vi "Configure Trigger Layer.vi"(0 "VISA resource name":refnum<visa-resource-name>, 1 "Trigger Count (1)":i32=1, 2 "Trigger Source (0: Auto-Internal)":i32(ring) items=["Auto-Internal", "EXT1", "EXT2", "EXT3", "EXT4", "EXT5", "EXT6", "EXT7", "LAN", "Internal Bus 1", "Internal Bus 2", "Bus", "Timer"], 3 "Timer Trigger Interval (1E-4 s)":dbl=0.0001, 5 "Channel (1: Channel 1)":i32(ring)=1 items=["Channel 1"=1, "Channel 2"=2], 7 "Device Action (2: Both)":i32(ring)=2 items=["Acquire", "Transient", "Both"], 9 "Bypass Setting (0: Off)":i32(ring) items=["Off", "Once"], 11 "error in (no error)":errorcluster, 12 "Trigger Delay (0 s)":dbl, 13 "LXI Triggers For Normal Trigger":bool[](array[boolean])=[TRUE, TRUE, TRUE, TRUE, TRUE, TRUE, TRUE, TRUE]) -> (4 "VISA resource name out":refnum<visa-resource-name>, 15 "error out":errorcluster)   [LabVIEW 2012, in "Keysight B2980 Series.lvlib"]
doc: "Configures the trigger layer in ARM-Trigger model."
uses:
  Keysight B2980 Series.lvlib
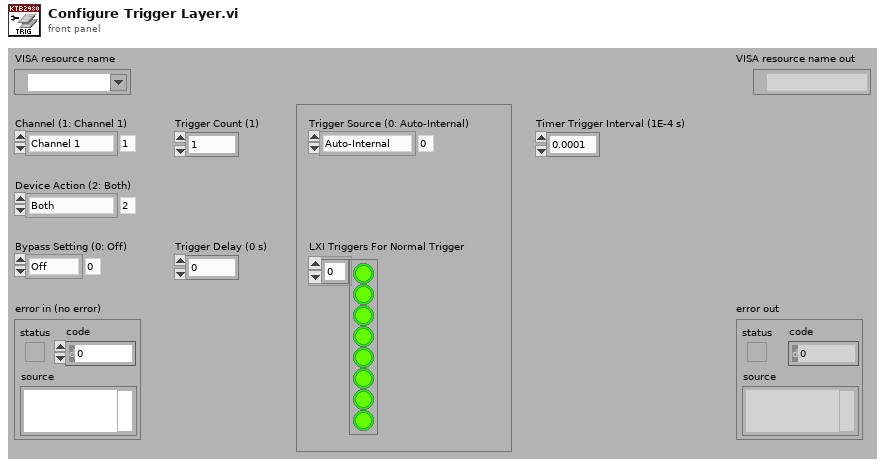
[diagram p1: front panel]
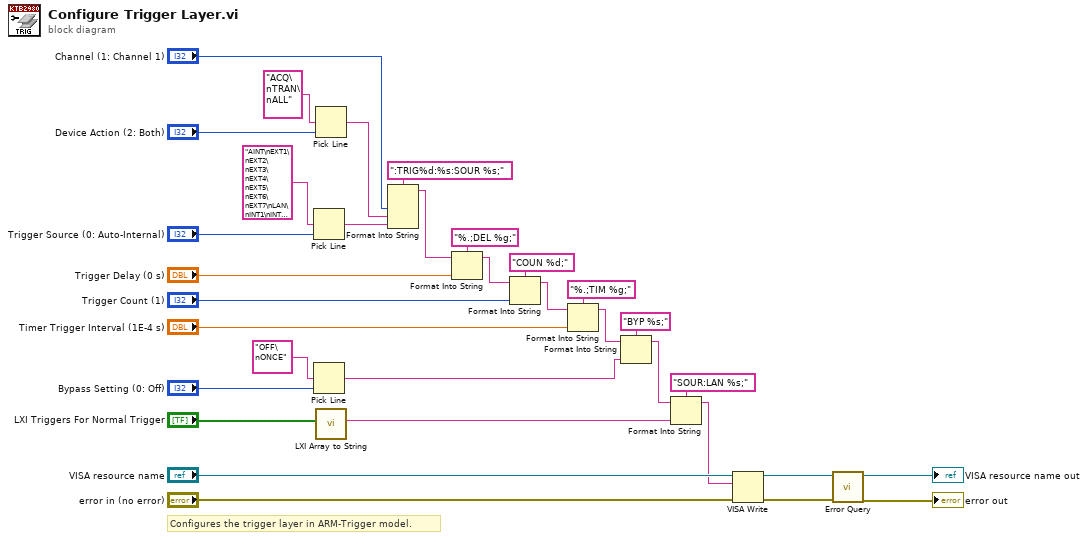
[diagram p0: block diagram]
diagram:
  # "Configures the trigger layer in ARM-Trigger model."
  n1 = Pick Line(multi-line string="AINT\nEXT1\nEXT2\nEXT3\nEXT4\nEXT5\nEXT6\nEXT7\nLAN\nINT1\nINT2\nBUS\nTIM", line index="Trigger Source (0: Auto-Internal)") -> (output string=w22:string)  [unwired: 1 out]
  n2 = Pick Line(multi-line string="OFF\nONCE", line index="Bypass Setting (0: Off)") -> (output string=w6:string)  [unwired: 1 out]
  n3 = Pick Line(multi-line string="ACQ\nTRAN\nALL", line index="Device Action (2: Both)") -> (output string=w13:string)  [unwired: 1 out]
  n4 = call "LXI Array to String.vi"("LXI Triggers"="LXI Triggers For Normal Trigger") -> ("LXI Command String"=w2:string)  [unwired: 10 out]
  n5 = Format Into String(format string=":TRIG%d:%s:SOUR %s;", "Channel (1: Channel 1)", w13, w22) -> (resulting string=w12:string)  [unwired: 2 in, 1 out]
  n6 = Format Into String(format string="%.;DEL %g;", initial string=w12, "Trigger Delay (0 s)") -> (resulting string=w10:string)  [unwired: 1 in, 1 out]
  n7 = Format Into String(format string="COUN %d;", initial string=w10, "Trigger Count (1)") -> (resulting string=w7:string)  [unwired: 1 in, 1 out]
  n8 = Format Into String(format string="%.;TIM %g;", initial string=w7, "Timer Trigger Interval (1E-4 s)") -> (resulting string=w5:string)  [unwired: 1 in, 1 out]
  n9 = Format Into String(format string="BYP %s;", initial string=w5, w6) -> (resulting string=w3:string)  [unwired: 1 in, 1 out]
  n10 = Format Into String(format string="SOUR:LAN %s;", initial string=w3, w2) -> (resulting string=w1:string)  [unwired: 1 in, 1 out]
  n11 = VISA Write(VISA resource name="VISA resource name", write buffer=w1, error in (no error)="error in (no error)") -> (VISA resource name out=w18:refnum<visa-resource-name>, error out=w17:errorcluster)  [unwired: 1 out]
  n12 = call "Error Query.vi"("error in (no error)"=w17, "VISA resource name"=w18) -> ("error out"=→"error out":errorcluster, "VISA resource name out"=→"VISA resource name out":refnum<visa-resource-name>)  [unwired: 8 out]
